vi "Pre Launch Init.vi"(11 "Nested in":refnum<class "UI Actor.lvclass">) -> (0 "error out":errorcluster, 3 "Nested out":refnum<class "UI Actor.lvclass">)   [LabVIEW 2020, in "UI Actor.lvlib" / "UI Actor.lvclass"]
doc: "(<B>Filename</B>: Actor Framework.lvlib:Actor.lvclass:Pre Launch Init.vi)\n\nDefines behavior that occurs after the Launch Nested Actor method is invoked but before the actor's Actor Core method begins running.\n\nBy default, this method does nothing. A descendant class may override it to define behavior."
uses:
  UI Actor.lvclass
  C:/Program Files/National Instruments/LabVIEW 2020/vi.lib/ActorFramework/Actor/Actor.lvclass
  UI Actor.lvclass/UI Actor.ctl
  <vilib>/ActorFramework/Actor/Actor.lvclass/Actor.ctl
  <vilib>/ActorFramework/Message Enqueuer/Message Enqueuer.lvclass/Message Enqueuer.ctl
  <vilib>/ActorFramework/Message Enqueuer/Init from Existing Queue.vi
  <vilib>/ActorFramework/Message Enqueuer/Enqueue.vi
  UI Actor Messages/VISA init Msg/VISA init Msg.lvclass
  C:/Program Files/National Instruments/LabVIEW 2020/vi.lib/ActorFramework/Message/Message.lvclass
  <vilib>/ActorFramework/Message Priority Queue/Priority Enqueue.vi
  <vilib>/ActorFramework/Message Enqueuer/Message Enqueuer.lvclass
  <vilib>/ActorFramework/Actor/Actor.lvclass
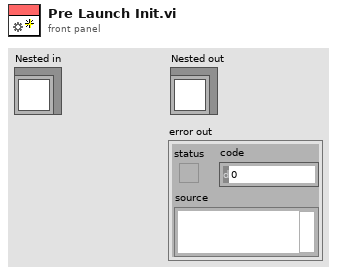
[diagram p1: front panel]
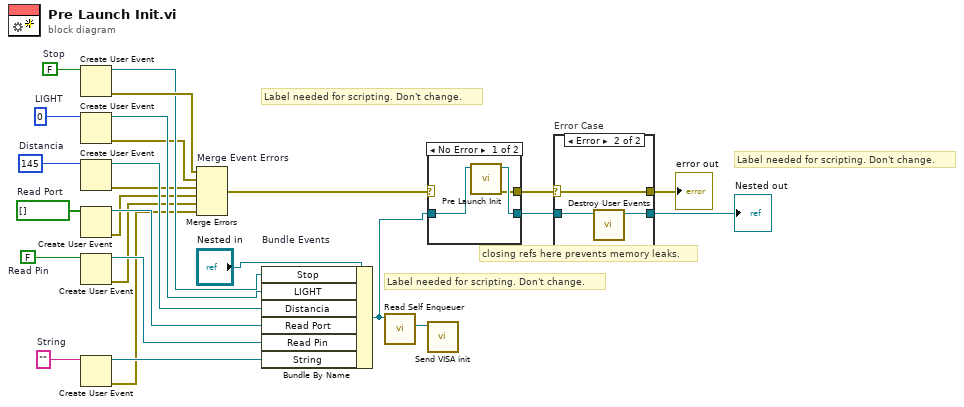
[diagram p0: block diagram]
diagram:
  w3 = ""  # String
  w8 = FALSE  # Read Pin
  w11 = bool[] []  # Read Port
  w14 = 145  # Distancia
  w17 = 0  # LIGHT
  w25 = FALSE  # Stop
  # "Label needed for scripting. Don't change."
  # "Label needed for scripting. Don't change."
  # "Label needed for scripting. Don't change."
  # "closing refs here prevents memory leaks."
  n1 = Create User Event(user event datatype=w25) -> (user event=w22:refnum<user-event>, error out=w24:errorcluster)  [unwired: 1 in]
  n2 = Create User Event(user event datatype=w17) -> (user event=w16:refnum<user-event>, error out=w15:errorcluster)  [unwired: 1 in]
  n3 = Create User Event(user event datatype=w14) -> (user event=w13:refnum<user-event>, error out=w12:errorcluster)  [unwired: 1 in]
  n4 = Create User Event(user event datatype=w11) -> (user event=w10:refnum<user-event>, error out=w9:errorcluster)  [unwired: 1 in]
  n5 = Create User Event(user event datatype=w8) -> (user event=w7:refnum<user-event>, error out=w6:errorcluster)  [unwired: 1 in]
  n6 = Create User Event(user event datatype=w3) -> (user event=w2:refnum<user-event>, error out=w1:errorcluster)  [unwired: 1 in]
  n7 = Merge Errors "Merge Event Errors"(w24, w15, w12, w9, w6, w1) -> (w19:errorcluster)
  n8 = Bundle By Name "Bundle Events"(cluster="Nested in", "Stop"=w22, "LIGHT"=w16, "Distancia"=w13, "Read Port"=w10, "Read Pin"=w7, "String"=w2) -> (w5:refnum<class "UI Actor.lvclass">)
  n9 = call <vilib>:"Read Self Enqueuer.vi"("Actor"=w5) -> ("Self Enqueuer"=w4:refnum<class "Message Enqueuer.lvclass">)  [unwired: 10 in]
  n10 = case shown="No Error" w19 {
    selector: w19 -> [_ w31]
    tunnel: [w29 w30] -> w20
    tunnel: w5 -> [w28 w30]
    tunnel: [w27 w31] -> w18
    frame No Error {
      n11 = call-parent "Pre Launch Init.vi"("Actor in"=w28) -> ("error out"=w27:errorcluster, "Actor out"=w29:refnum<class "UI Actor.lvclass">)  [unwired: 9 in]
    }
    frame Error {
    }
  }
  n12 = call "Send VISA init.vi"("Message Enqueuer"=w4) -> ()  [unwired: 9 in, 2 out]
  n13 = case "Error Case" shown="Error" w18 {
    selector: w18 -> [w32 w36]
    tunnel: w20 -> [w33 w35]
    tunnel: [w33 w34] -> w23
    tunnel: [w32 w36] -> w21
    frame No Error {
    }
    frame Error {
      n14 = call "Destroy User Events.vi"("UI Template in"=w35) -> ("UI Template out"=w34:refnum<class "UI Actor.lvclass">)  [unwired: 10 in]
    }
  }
  "error out" <- w21
  "Nested out" <- w23
